vi "decoupling.vi"(9 "Input":sgl[](array[numeric])) -> (1 "Output":sgl[](array[numeric]))   [LabVIEW 2013]
uses:
  <vilib>/Analysis/baseanly.llb/A x Vector.vi
  decoupling_global.vi
  <vilib>/Analysis/NI_AALBase.lvlib
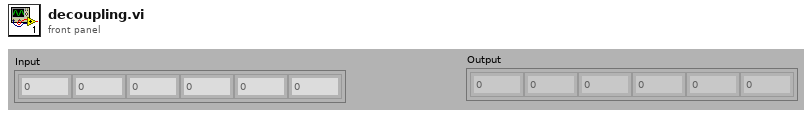
[diagram p1: front panel]
types:
  T1 = typedef "NI_Matrix.lvlib/RealMatrix.ctl" = dbl[][]
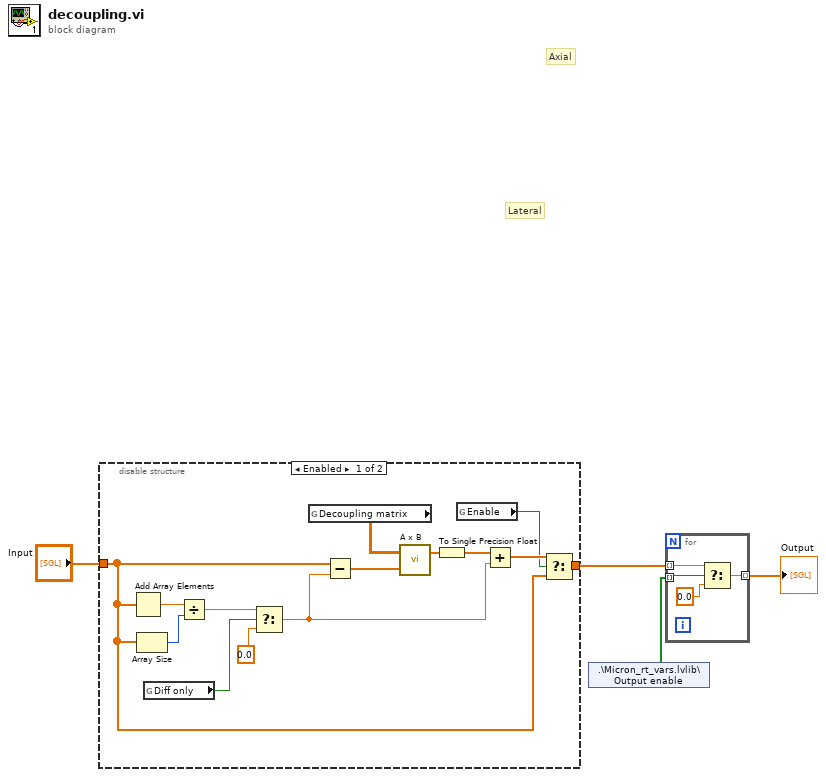
[diagram p0: block diagram]
diagram:
  # "Axial"
  # "Lateral"
  n1 = disable-structure shown="Enabled" {
    disable-tunnel: "Input" -> [w6 w19]
    disable-tunnel: [w5 w19] -> w3
    frame Enabled {
      n2 = Add Array Elements(numeric array=w6) -> (sum=w16:sgl)
      n3 = Array Size(array=w6) -> (size(s)=w15:i32)
      n4 = global read "decoupling_global.vi" "Diff only"() -> (w10:bool)
      n5 = Divide(x=w16, y=w15) -> (x/y=w12:sgl)
      n6 = Select(t=w12, s=w10, f=sgl 0.0) -> (s? t:f=w11:sgl)
      n7 = global read "decoupling_global.vi" "Decoupling matrix"() -> (w18:T1)
      n8 = Subtract(x=w6, y=w11) -> (x-y=w14:sgl[])
      n9 = call-poly <vilib>:"A x B.vi"("Vector"=w14, "A"=w18) -> ("A x Vector"=w17:dbl[])  [unwired: 1 out]
      n10 = To Single Precision Float(number=w17) -> (single precision float=w13:sgl[])
      n11 = global read "decoupling_global.vi" "Enable"() -> (w7:bool)
      n12 = Add(x=w13, y=w11) -> (x+y=w8:sgl[])
      n13 = Select(t=w8, s=w7, f=w6) -> (s? t:f=w5:sgl[])
    }
    frame Disabled {
    }
  }
  n14 = shared-variable ".\\Micron_rt_vars.lvlib\\Output enable"() -> (w4:bool[])  [unwired: 1 in, 1 out]
  n15 = for {
    tunnel: w3 -> [w23] mode=indexing
    tunnel: w4 -> [w20] mode=indexing
    tunnel: [w21] -> w1 mode=indexing
    n16 = Select(t=w23, s=w20, f=sgl 0.0) -> (s? t:f=w21:sgl)
  }
  "Output" <- w1
